vi "SPI_FPGA_Top_Level_Main.vi"(5 "FPGA IO":T1={"SCLK"="DIO18", "CS_1"="DIO16", "MOSI"="DIO26", "MISO"="DIO25"}) -> ()   [LabVIEW 2012]
uses:
  Controls/FPGA SPI_Cmd.ctl
  <vilib>/Platform/TimedLoop/XDataNode/timing_clust.ctl
  <vilib>/Platform/TimedLoop/XDataNode/nitl_modes.ctl
  <vilib>/Platform/TimedLoop/XDataNode/wakeup.ctl
  Controls/FPGA SPI_Arb Loop State.ctl
  <vilib>/rvi/Emulation/niFpgaSctlEmulationRegisterWithScheduler.vi
  <vilib>/rvi/eio/common/nirviEmuTemplateMethod_errors.vi
  <vilib>/rvi/Emulation/niFpgaSctlEmulationScheduler.vi
  <vilib>/rvi/Emulation/niFpgaSctlEmulationGetInTimedLoop.vi
  Code/FPGA SPI_Globals.vi
  <vilib>/rvi/Emulation/niFpgaSctlEmulationGlobalWrite.vi
  <vilib>/rvi/DataTransferAndStorage/Container/Common/niFpgaContainerGetUniqueNameForEmu.vi
  <vilib>/rvi/FIFO/Fifo_Resource/nirvififoEmulationSetSize.vi
  <vilib>/rvi/errors/niFpgaSetErrorForExecOnDevCompSimple.vi
  <vilib>/rvi/eio/common/nirviEmuReportErrorAndStop.vi
  <vilib>/rvi/Emulation/niFpgaSctlEmulationFifoFullMgr.vi
  <vilib>/rvi/Emulation/niFpgaSctlEmulationResourceMgr.vi
  <vilib>/platform/TimedLoop/XDataNode/XDataNode.xnode
  <vilib>/eio/EIOMethodNode/EIOMethodNode.xnode
  <vilib>/eio/EIONode/EIONode.xnode
  <vilib>/rvi/DataTransferAndStorage/Container/XNode/niFpgaContainer.xnode
  <vilib>/rvi/FIFO/Fifo_Resource/nirvififoEmulationWrite.vi
  <vilib>/rvi/FIFO/Fifo_Resource/nirvififoEmulationRead.vi
  <vilib>/Platform/TimedLoop/XDataNode/XDNodeRunTimeDep.lvlib
panel:
  in  "SPI_READ?":bool
  out "Ready":bool
  in  "SPI_Clock Divider":u32=20
  in  "SPI_CS Active State":bool caption="SPI_CS\nActive State"
  in  "SPI_CPOL":bool
  in  "SPI_CPHA":bool
  in  "SPI_CS":u8=1 format="%08b"
  in  "SPI_Total Bits":u16=8
  in  "SPI_Total Bytes":u16=1
  in  "SPI_Start":bool
  in  "SPI_Cmd":T2=enum."Configure"
  in  "SPI_Ack Read":bool
  out "SPI_Read Data":u8
  out "SPI_Read Flag":bool
  in  "SPI_Write Flag":bool
  in  "SPI_Write Data":u8
  in  "SPI_Port":u8
  # "Control"
  # "SPI Configuration Parameters"
  # "Command Type"
  # "Host Data Transfer"
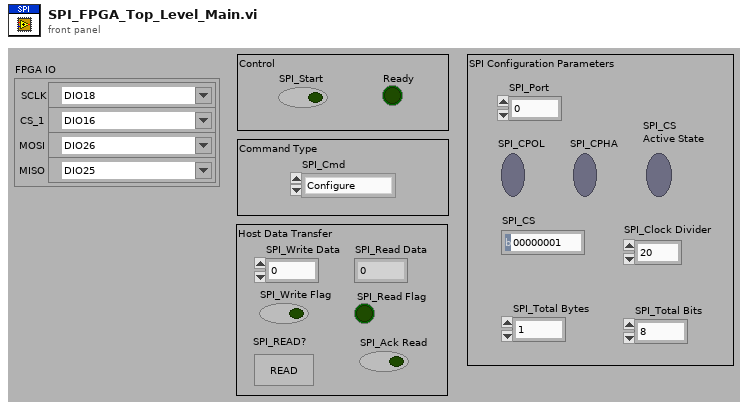
[diagram p1: front panel]
types:
  T1 = cluster{"SCLK":refnum<k21>, "CS_1":refnum<k21>, "MOSI":refnum<k21>, "MISO":refnum<k21>}
  T2 = typedef "FPGA SPI_Cmd.ctl" = enum8{"Idle", "Write/Read SPI", "Configure"}
  T3 = typedef "XDNodeRunTimeDep.lvlib/timing_clust.ctl" = cluster{"Expected End [f-1]":u64, "Actual End [f-1]":u64, "Finished Late? [f-1]":bool, "Expected End [i-1]":u64, "Actual End [i-1]":u64, "Finished Late? [i-1]":bool, "Expected Start [i]":u64, "Actual Start [i]":u64, "Expected Start [f]":u64, "Actual Start [f]":u64, "Source Name":string, "Structure Name":string, "Period":i64, "Deadline":i64, "Offset":i64, "Start":i64, "Priority":i32, "Timeout":i32, "Mode":T4, "Wakeup Reason":T5, "Error":errorcluster, "Source Type":string, "Secondary Source Type":string, "Global End Time":u64, "Global Start Time":u64, "Frame Duration":u64, "Iteration Duration":u64, "Assigned CPU":i32, "I/O Scan Engine Mode":u32}
  T4 = typedef "XDNodeRunTimeDep.lvlib/nitl_modes.ctl" = enum32{"No Change", "Process missed periods, maintain original phase", "Discard missed periods, maintain original phase", "Process missed periods, ignore original phase", "Discard missed periods, ignore original phase"}
  T5 = typedef "XDNodeRunTimeDep.lvlib/wakeup.ctl" = enum32{"Normal", "Aborted", "Asynchronous wakeup", "Timing source error", "Timed loop error", "Timeout"}
  T6 = enum16{"high", "wait", "low", "wait low", "high_2", "end"}
  T7 = typedef "FPGA SPI_Arb Loop State.ctl" = enum8{"Idle", "Init", "Write", "Start", "Read", "Wait Until Done"}
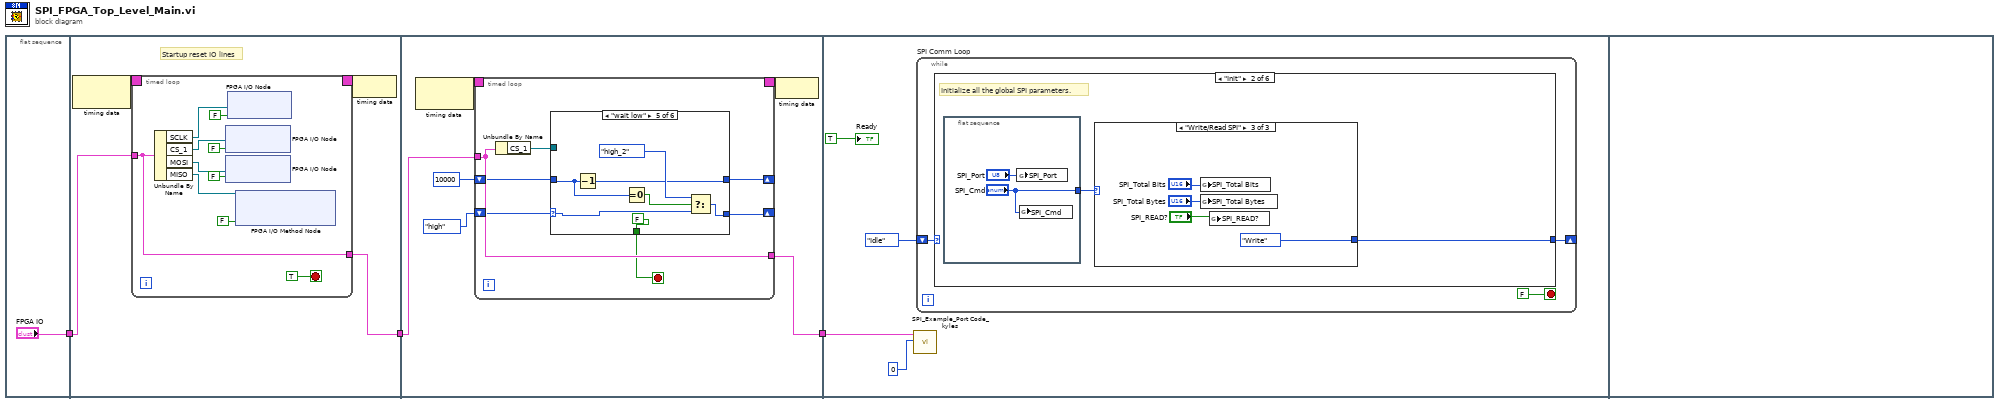
[diagram p0: block diagram]
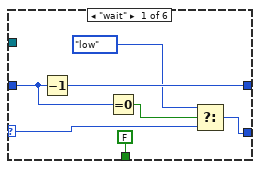
[diagram p2: hidden frame]
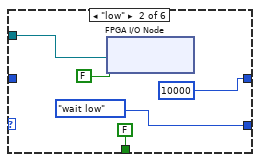
[diagram p3: hidden frame]
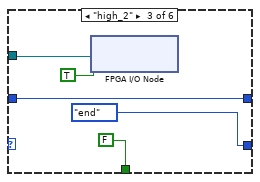
[diagram p4: hidden frame]
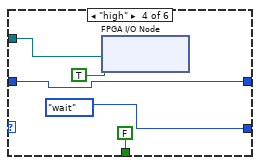
[diagram p5: hidden frame]
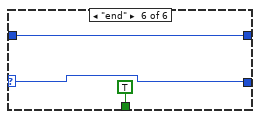
[diagram p6: hidden frame]
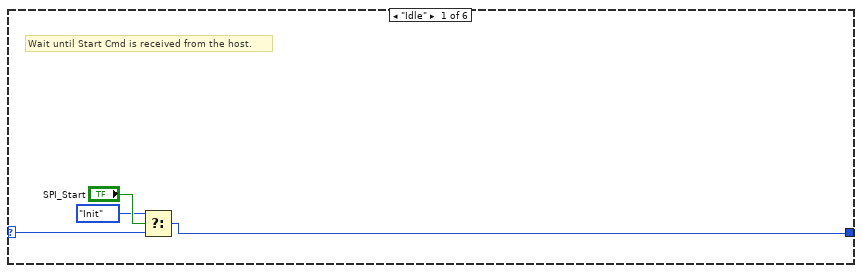
[diagram p7: hidden frame]
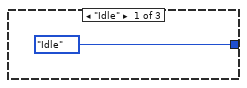
[diagram p8: hidden frame]
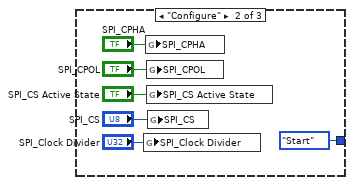
[diagram p9: hidden frame]
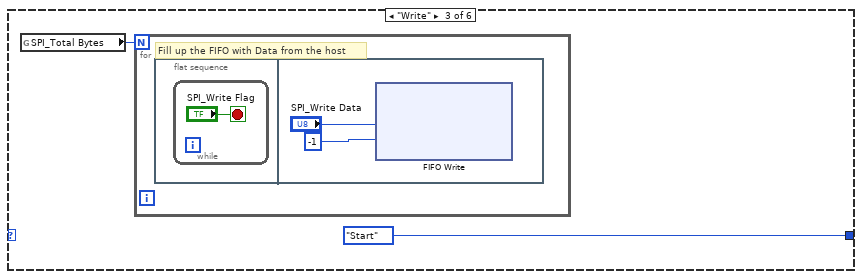
[diagram p10: hidden frame]
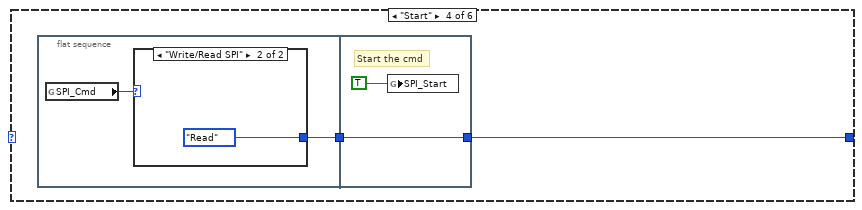
[diagram p11: hidden frame]
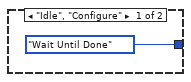
[diagram p12: hidden frame]
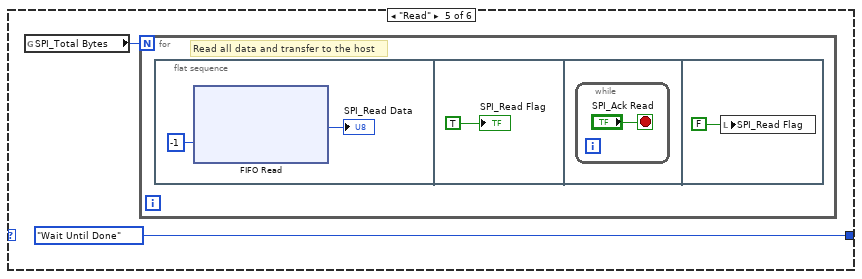
[diagram p13: hidden frame]
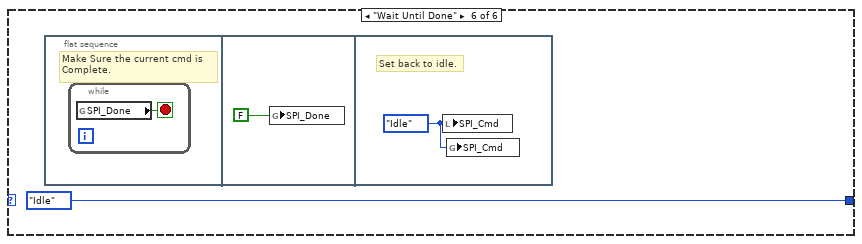
[diagram p14: hidden frame]
diagram:
  n1 = flat-sequence {
    tunnel: ["FPGA IO"] -> w3
    tunnel: w3 -> [w6]
    tunnel: [w5] -> w2
    tunnel: w2 -> [w26]
    tunnel: [w25] -> w1
    tunnel: w1 -> [w72]
    frame #0 {
    }
    frame #1 {
      # "Startup reset IO lines"
      n2 = node-c288() -> (w8:T3)  [unwired: 1 in]
      n3 = timed-loop {
        timing: w8 -> [_]
        timing-out: [_] -> w7
        tunnel: w6 -> [w17]
        tunnel: [w17] -> w5
        stop <- TRUE stop-if-true
        n4 = Unbundle By Name(w17) -> ("SCLK"=w16:refnum<k21>, "CS_1"=w15:refnum<k21>, "MOSI"=w14:refnum<k21>, "MISO"=w13:refnum<k21>)
        n5 = xnode "FPGA I/O Node"("I/O Item"=FALSE, "FPGA I/O In"=w15) -> ()  [unwired: 1 out]
        n6 = xnode "FPGA I/O Node"("I/O Item"=FALSE, "FPGA I/O In"=w14) -> ()  [unwired: 1 out]
        n7 = xnode "FPGA I/O Node"("I/O Item"=FALSE, "FPGA I/O In"=w16) -> ()  [unwired: 1 out]
        n8 = xnode "FPGA I/O Method Node"("FPGA I/O In"=w13, "Enable"=FALSE) -> ()  [unwired: 1 out]
      }
      n9 = node-c288(w7) -> ()
    }
    frame #2 {
      n10 = node-c288() -> (w28:T3)  [unwired: 1 in]
      n11 = timed-loop {
        timing: w28 -> [_]
        timing-out: [_] -> w27
        tunnel: w26 -> [w35]
        tunnel: [w35] -> w25
        shift-right: [w33] -> _
        shift-left: T6."high" -> [w32]
        shift-right: [w29] -> _
        shift-left: i16 10000 -> [w30]
        stop <- w31 stop-if-true
        n12 = Unbundle By Name(w35) -> ("CS_1"=w34:refnum<k21>)
        n13 = case shown="\"wait low\"" w32 {
          selector: w32 -> [w41 _ _ _ w60 w65]
          tunnel: w34 -> [_ w46 w49 w56 _ _]
          tunnel: [w40 T6."wait low" T6."end" T6."wait" w58 w65] -> w33
          tunnel: [FALSE FALSE FALSE FALSE FALSE TRUE] -> w31
          tunnel: w30 -> [w37 _ w51 w54 w61 w66]
          tunnel: [w39 i16 10000 w51 w54 w62 w66] -> w29
          frame "wait" {
            n14 = Decrement(x=w37) -> (x-1=w39:i16)
            n15 = Equal To 0?(x=w37) -> (x = 0?=w38:bool)
            n16 = Select(t=T6."low", s=w38, f=w41) -> (s? t:f=w40:T6)
          }
          frame "low" {
            n17 = xnode "FPGA I/O Node"("I/O Item"=FALSE, "FPGA I/O In"=w46) -> ()  [unwired: 1 out]
          }
          frame "high_2" {
            n18 = xnode "FPGA I/O Node"("I/O Item"=TRUE, "FPGA I/O In"=w49) -> ()  [unwired: 1 out]
          }
          frame "high" {
            n19 = xnode "FPGA I/O Node"("I/O Item"=TRUE, "FPGA I/O In"=w56) -> ()  [unwired: 1 out]
          }
          frame "wait low" {
            n20 = Decrement(x=w61) -> (x-1=w62:i16)
            n21 = Equal To 0?(x=w61) -> (x = 0?=w63:bool)
            n22 = Select(t=T6."high_2", s=w63, f=w60) -> (s? t:f=w58:T6)
          }
          frame "end" {
          }
        }
      }
      n23 = node-c288(w27) -> ()
    }
    frame #3 {
      n24 = call "SPI_Example_Port Code_kyles.vi"("Port"=i8 0, "FPGA IO"=w72) -> ()  [unwired: 10 in]
      n25 = while "SPI Comm Loop" {
        shift-right: [w77] -> _
        shift-left: FPGA_SPI_Arb_Loop_State."Idle" ("Action") -> [w76]
        stop <- FALSE stop-if-true
        n26 = case shown="\"Init\"" w76 {
          selector: w76 -> [w81 _ _ _ _ _]
          tunnel: [w79 w83 FPGA_SPI_Arb_Loop_State."Start" ("Action") w104 FPGA_SPI_Arb_Loop_State."Wait Until Done" ("Action") FPGA_SPI_Arb_Loop_State."Idle" ("Action")] -> w77
          frame "Idle" {
            # "Wait until Start Cmd is received from the host."
            n27 = Select(t=FPGA_SPI_Arb_Loop_State."Init" ("Action"), s="SPI_Start", f=w81) -> (s? t:f=w79:T7)
          }
          frame "Init" {
            # "Initialize all the global SPI parameters."
            n28 = flat-sequence {
              tunnel: ["SPI_Cmd"] -> w84
              frame #0 {
                n29 = global write "FPGA SPI_Globals.vi" "SPI_Port"("SPI_Port") -> ()
                n30 = global write "FPGA SPI_Globals.vi" "SPI_Cmd"("SPI_Cmd") -> ()
              }
            }
            n31 = case shown="\"Write/Read SPI\"" w84 {
              tunnel: [FPGA_SPI_Arb_Loop_State."Idle" ("Action") FPGA_SPI_Arb_Loop_State."Start" ("Action") FPGA_SPI_Arb_Loop_State."Write" ("Action")] -> w83
              frame "Idle" {
              }
              frame "Configure" {
                n32 = global write "FPGA SPI_Globals.vi" "SPI_Clock Divider"("SPI_Clock Divider") -> ()
                n33 = global write "FPGA SPI_Globals.vi" "SPI_CPHA"("SPI_CPHA") -> ()
                n34 = global write "FPGA SPI_Globals.vi" "SPI_CPOL"("SPI_CPOL") -> ()
                n35 = global write "FPGA SPI_Globals.vi" "SPI_CS Active State"("SPI_CS Active State") -> ()
                n36 = global write "FPGA SPI_Globals.vi" "SPI_CS"("SPI_CS") -> ()
              }
              frame "Write/Read SPI" {
                n37 = global write "FPGA SPI_Globals.vi" "SPI_Total Bits"("SPI_Total Bits") -> ()
                n38 = global write "FPGA SPI_Globals.vi" "SPI_Total Bytes"("SPI_Total Bytes") -> ()
                n39 = global write "FPGA SPI_Globals.vi" "SPI_READ?"("SPI_READ?") -> ()
              }
            }
          }
          frame "Write" {
            n40 = global read "FPGA SPI_Globals.vi" "SPI_Total Bytes"() -> (w99:u16)
            n41 = for {
              N: w99 -> [_]
              # "Fill up the FIFO with Data from the host"
              n42 = flat-sequence {
                frame #0 {
                  n43 = while {
                    stop <- "SPI_Write Flag" stop-if-true
                  }
                }
                frame #1 {
                  n44 = xnode ("FIFO Write")("Element"="SPI_Write Data", "Timeout"=-1) -> ()  [unwired: 1 in, 2 out]
                }
              }
            }
          }
          frame "Start" {
            n45 = flat-sequence {
              tunnel: [w105] -> w103
              tunnel: [w110] -> w104
              tunnel: w103 -> [w110]
              frame #0 {
                n46 = global read "FPGA SPI_Globals.vi" "SPI_Cmd"() -> (w106:T2)
                n47 = case shown="\"Write/Read SPI\"" w106 {
                  tunnel: [FPGA_SPI_Arb_Loop_State."Wait Until Done" ("Action") FPGA_SPI_Arb_Loop_State."Read" ("Action")] -> w105
                  frame "Idle", "Configure" {
                  }
                  frame "Write/Read SPI" {
                  }
                }
              }
              frame #1 {
                # "Start the cmd"
                n48 = global write "FPGA SPI_Globals.vi" "SPI_Start"(TRUE ("Write Flag")) -> ()
              }
            }
          }
          frame "Read" {
            n49 = global read "FPGA SPI_Globals.vi" "SPI_Total Bytes"() -> (w112:u16)
            n50 = for {
              N: w112 -> [_]
              # "Read all data and transfer to the host"
              n51 = flat-sequence {
                frame #0 {
                  n52 = xnode ("FIFO Read")("Timeout"=-1) -> ("Element"=→"SPI_Read Data":u8)  [unwired: 1 in, 2 out]
                }
                frame #1 {
                  "SPI_Read Flag" <- TRUE ("Read Flag")
                }
                frame #2 {
                  n53 = while {
                    stop <- "SPI_Ack Read" stop-if-true
                  }
                }
                frame #3 {
                  n54 = local write "SPI_Read Flag"(FALSE ("Read Flag")) -> ()
                }
              }
            }
          }
          frame "Wait Until Done" {
            n55 = flat-sequence {
              frame #0 {
                # "Make Sure the current cmd is\nComplete."
                n56 = while {
                  stop <- w119 stop-if-true
                  n57 = global read "FPGA SPI_Globals.vi" "SPI_Done"() -> (w119:bool)
                }
              }
              frame #1 {
                n58 = global write "FPGA SPI_Globals.vi" "SPI_Done"(FALSE ("Done")) -> ()
              }
              frame #2 {
                w121 = FPGA_SPI_Cmd."Idle" ("Type")
                # "Set back to idle."
                n59 = local write "SPI_Cmd"(w121) -> ()
                n60 = global write "FPGA SPI_Globals.vi" "SPI_Cmd"(w121) -> ()
              }
            }
          }
        }
      }
      "Ready" <- TRUE ("Ready")
    }
    frame #4 {
    }
  }
